vi "1C Camera - Mask Pool Edge.vi"(10 "Pool Oval ROI":T1={"Global Rectangle"=[69, -100, 1339, 1142], "Contours"=[{"Contour Type"=0, "ROI Type"=4, "Points"=[69, -100, 1339, 1142]}]}, 11 "Source Image In":T2) -> (2 "Masked Image Out":T2, 3 "Src Image Out":T2)   [LabVIEW 2011]
doc: "Creates a copy of the source image, with everything outside the pool removed. On the original image, overlays an oval depicting the pool edge.\n\nPurpose: Removing extraneous objects from the image will increase reliability of our pattern matching algorithm.\n\nBy: Jason Curtis, Nov 17 2011"
uses:
  <vilib>/vision/Image Controls.llb/IMAQ Image.ctl
  <vilib>/vision/NI_Vision_Development_Module.lvlib
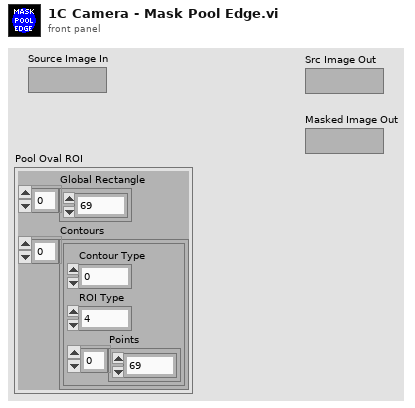
[diagram p1: front panel]
types:
  T1 = cluster{"Global Rectangle":i32[], "Contours":cluster{"Contour Type":u32, "ROI Type":u32, "Points":i32[]}[]}
  T2 = typedef "IMAQ Image.ctl" = refnum<image>
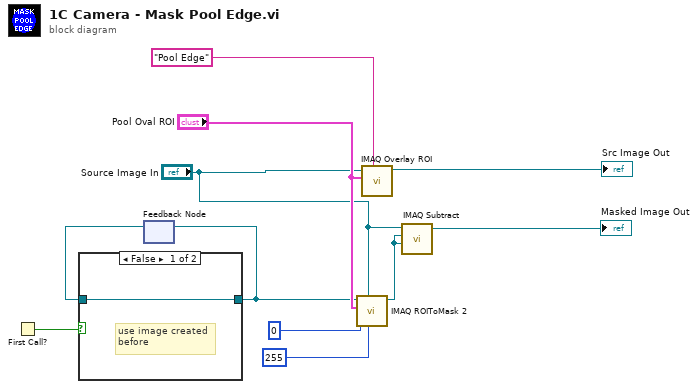
[diagram p0: block diagram]
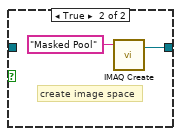
[diagram p2: hidden frame]
diagram:
  n1 = First Call?() -> (First Call?: T/F=w5:bool)
  n2 = feedback #1() -> (w3:T2)  [unwired: 1 in]
  n3 = case shown="False" w5 {
    tunnel: [w12 w14] -> w4
    tunnel: w3 -> [w12 _]
    frame False {
      # "use image created\nbefore"
    }
    frame True {
      # "create image space"
      n4 = call "IMAQ Create"("Image Name"="Masked Pool") -> ("New Image"=w14:T2)  [unwired: 4 in, 1 out]
    }
  }
  n5 = feedback-in #1(w4) -> ()
  n6 = call "IMAQ ROIToMask 2"("Background Value (0)"=255, "Image Model"="Source Image In", "Filling Value (255)"=0, "ROI Descriptor"="Pool Oval ROI", "Image"=w4) -> ("Image Out"=w8:T2)  [unwired: 4 in, 2 out]
  n7 = call "IMAQ Overlay ROI"("Group"="Pool Edge", "ROI Descriptor"="Pool Oval ROI", "Image"="Source Image In") -> ("Image Out"=→"Src Image Out":T2)  [unwired: 7 in, 1 out]
  n8 = call "IMAQ Subtract"("Image Src A"="Source Image In", "Image Dst"=w8, "Image Src B"=w8) -> ("Image Dst Out"=→"Masked Image Out":T2)  [unwired: 2 in, 3 out]
